vi "NI VeriStand - Set Multiple Faults.vi"(8 "error in (no error)":errorcluster, 9 "Fault Values":dbl[](array[numeric]), 10 "Channels":string[](array[string]), 11 "ChannelFault in":T1) -> (0 "error out":errorcluster, 3 "ChannelFault out":T1)   [LabVIEW 2020, in "NI_VS ChannelFault ExecutionAPI.lvlib"]
doc: "Sets the fault value for all specified channels."
uses:
  <vilib>/NI VeriStand/Execution/ChannelFaultManager/NI_VS ChannelFault ExecutionAPI.lvlib
  <vilib>/NI VeriStand/Execution/ChannelFaultManager/ChannelFaultAPI.ctl
  NationalInstruments.VeriStand.ClientAPI
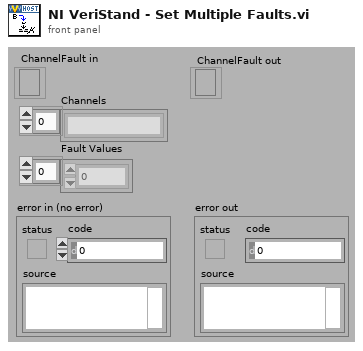
[diagram p1: front panel]
types:
  T1 = typedef "NI_VS ChannelFault ExecutionAPI.lvlib/ChannelFaultAPI.ctl" = refnum<k24>
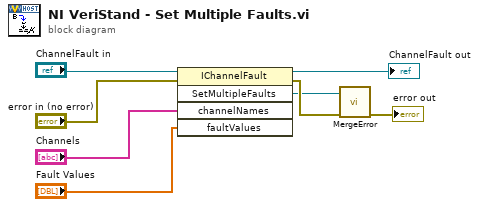
[diagram p0: block diagram]
diagram:
  n1 = invoke class="IChannelFault" method="SetMultipleFaults"(reference="ChannelFault in", error in="error in (no error)", "channelNames"="Channels", "faultValues"="Fault Values") -> (reference out=→"ChannelFault out":T1, error out=w6:errorcluster, "SetMultipleFaults"=w5:refnum<k24>)  [unwired: 1 in, 2 out]
  n2 = call <vilib>:"MergeError.vi"("error in (no error)"=w6, "Error"=w5) -> ("error out"=→"error out":errorcluster)  [unwired: 9 out]
